vi "Plug_in_Alberto.vi"() -> (5 "Plug in titles":string[](array[string]), 7 "Plug in values":string[](array[string]))   [LabVIEW 2010]
uses:
  Globals/Meas_global.vi
  Globals/Plug_in_data_global.vi
panel:
  out "Appended path name":path
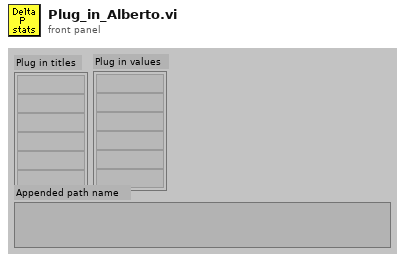
[diagram p1: front panel]
types:
  T1 = cluster{"Name":string, "X":dbl, "Y":dbl, "Z":dbl}[]
  T2 = cluster{"Name":string, "X":dbl, "Y":dbl, "Z":dbl}
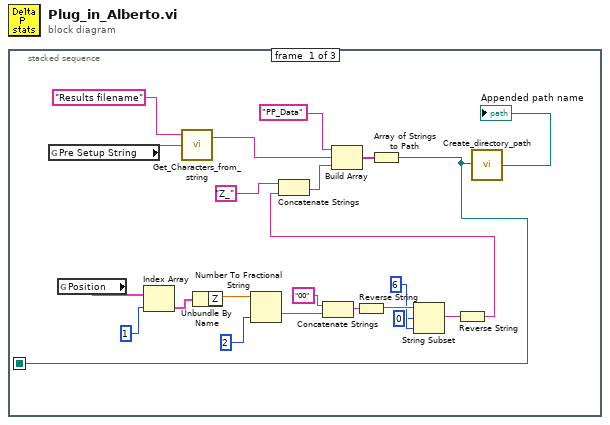
[diagram p0: block diagram]
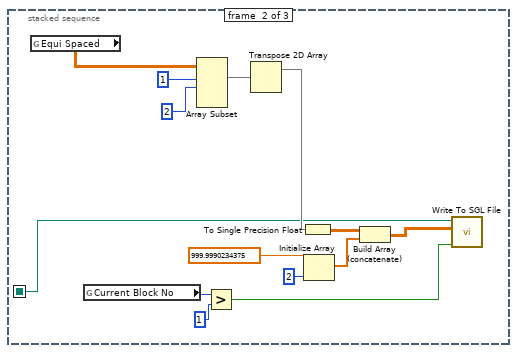
[diagram p2: hidden frame]
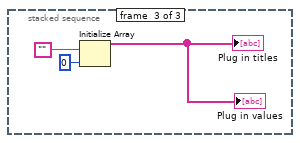
[diagram p3: hidden frame]
diagram:
  n1 = stacked-sequence {
    seq-local: [w1 _ _] -> [_ w31 _]
    frame #0 {
      n2 = global read "Meas_global.vi" "Pre Setup String"() -> (w22:string)
      n3 = global read "Meas_global.vi" "Position"() -> (w20:T1)
      n4 = Index Array(array=w20, index=1 ("Index")) -> (element=w18:T2)
      n5 = call "Get_Characters_from_string.vi"("Input string"=w22, "Variable name"="Results filename") -> ("Value"=w4:string)  [unwired: 1 in, 1 out]
      n6 = Unbundle By Name(w18) -> ("Z"=w17:dbl)
      n7 = Number To Fractional String(number=w17, precision (6)=i16 2) -> (F-format string=w15:string)  [unwired: 2 in]
      n8 = Concatenate Strings("00" ("Substring"), w15) -> (w13:string)
      n9 = Reverse String(1:w13) -> (0:w12:string)
      n10 = String Subset(string=w12, offset (0)=0, length (rest)=6 ("length")) -> (substring=w9:string)
      n11 = Reverse String(1:w9) -> (0:w8:string)
      n12 = Concatenate Strings("Z_" ("Substring"), w8) -> (w3:string)
      n13 = Build Array("PP_Data" ("Substring"), w4, w3) -> (w2:string[])
      n14 = Array of Strings to Path(0:w2) -> (2:w1:path)  [unwired: 1 in]
      n15 = call "Create_directory_path.vi"("Path name"=w1) -> ("Path name Out"=→"Appended path name":path)
    }
    frame #1 {
      n16 = global read "Plug_in_data_global.vi" "Equi Spaced"() -> (w36:dbl[][])
      n17 = global read "Meas_global.vi" "Current Block No"() -> (w25:i32)
      n18 = Array Subset(array=w36, index (row)=1 ("Array Index"), length (row)=2 ("Array Length")) -> (w33:dbl[][])  [unwired: 2 in]
      n19 = Greater?(x=w25, y=1) -> (0:w23:bool)
      n20 = Transpose 2D Array(2D array=w33) -> (transposed array=w32:dbl[][])
      n21 = To Single Precision Float(number=w32) -> (single precision float=w30:sgl[][])
      n22 = Initialize Array(sgl 999.999, 2 ("Dimension Size")) -> (w29:sgl[])
      n23 = Build Array (concatenate)(w30, w29) -> (w26:sgl[][])
      n24 = call <vilib>:"Write To SGL File.vi"("append to file? (new file:F)"=w23, "2D array"=w26, "file path (dialog if empty)"=w31) -> ()  [unwired: 4 in, 1 out]
    }
    frame #2 {
      n25 = Initialize Array("", 0) -> (→"Plug in titles" →"Plug in values":string[])
    }
  }
